vi "Test DAQmx Digitizer.vi"() -> ()   [LabVIEW 2015]
uses:
  Instruments/Pulse Driver/Pusle Driver Configuration.ctl
  DAQmx Digitizer.lvclass
  Instruments/Pulse Driver/Pulse Driver.lvclass/Pulse Driver.ctl
  Instruments/Pulse Driver/Write tdms file.vi
  Instruments/Pulse Driver/Write User Configuration.vi
panel:
  in  "User Configuration":T1={"Pre-trigger duration"=0.01, "Post-trigger duration"=0.1, "Rate"=1000000.0, "Ranges"=[10.0], "Re-name channels"=[], "Active channels"="0:1", "External clock"=FALSE} {"Rate" format="%#_6pHz"; "Post-trigger duration" format="%#_6ps"; "Pre-trigger duration" format="%#_6ps"; "Ranges" format="%#_6pV"}
  in  "File Path Control":path=path "D:/Data/test_daqmx.tdms"
  in  "Stop Button":bool
  out "Availiable Samples":u32=110000
  out "Finished":bool=TRUE
  out "Armed":bool
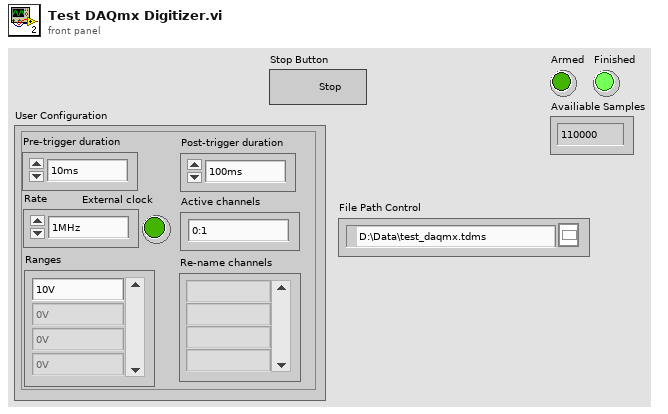
[diagram p1: front panel]
types:
  T1 = typedef "Pusle Driver Configuration.ctl" = cluster{"Pre-trigger duration":dbl, "Post-trigger duration":dbl, "Rate":dbl, "Ranges":dbl[], "Re-name channels":string[], "Active channels":string, "External clock":bool}
  T2 = enum16{"open", "open or create", "create or replace", "create", "open (read-only)"}
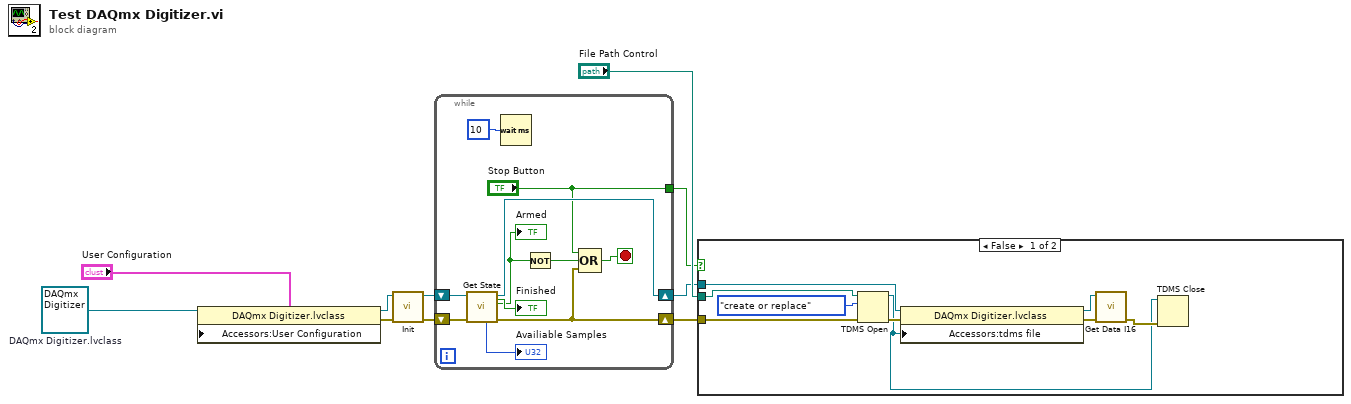
[diagram p0: block diagram]
diagram:
  w10 = refnum<class "DAQmx Digitizer.lvclass"> refnum  # DAQmx Digitizer.lvclass
  n1 = property class="DAQmx Digitizer.lvclass"(reference=w10, "Accessors:User Configuration"="User Configuration") -> (reference out=w9:refnum<class "DAQmx Digitizer.lvclass">, error out=w8:errorcluster)  [unwired: 1 in]
  n2 = call-dynamic "Init.vi"("error in (no error)"=w8, "Pulse Driver in"=w9) -> ("error out"=w6:errorcluster, "Pulse Driver out"=w7:refnum<class "DAQmx Digitizer.lvclass">)  [unwired: 8 in]
  n3 = while {
    shift-right: [w11] -> w5
    shift-left: w6 -> [w20]
    shift-right: [w13] -> w3
    shift-left: w7 -> [w21]
    tunnel: ["Stop Button"] -> w2
    stop <- w16 stop-if-true
    n4 = call-dynamic "Get State.vi"("error in (no error)"=w20, "DAQmx Digitizer in"=w21) -> ("error out"=w11:errorcluster, "Armed"=w15:bool, "DAQmx Digitizer out"=w13:refnum<class "DAQmx Digitizer.lvclass">, "Availiable Samples"=→"Availiable Samples":u32, "Finished"=→"Finished":bool)  [unwired: 4 in, 1 out]
    "Armed" <- w15
    n5 = Wait (ms)(milliseconds to wait=u32 10) -> ()  [unwired: 1 out]
    n6 = Not(x=w15) -> (.not. x?=w14:bool)
    n7 = Compound Arithmetic op=OR("Stop Button", w14, w11) -> (w16:bool)
  }
  n8 = case shown="False" w2 {
    tunnel: w5 -> [w30 _]
    tunnel: "File Path Control" -> [w29 _]
    tunnel: w3 -> [w27 _]
    frame False {
      n9 = TDMS Open(8:w30, 10:T2."create or replace" ("operation (0:open)"), 11:w29) -> (0:w25:errorcluster, 3:w22:refnum<k34>)  [unwired: 4 in]
      n10 = property class="DAQmx Digitizer.lvclass"(reference=w27, error in=w25, "Accessors:tdms file"=w22) -> (reference out=w26:refnum<class "DAQmx Digitizer.lvclass">, error out=w24:errorcluster)
      n11 = call-dynamic "Get Data I16.vi"("error in (no error)"=w24, "DAQmx Digitizer in"=w26) -> ("error out"=w23:errorcluster)  [unwired: 5 in, 4 out]
      n12 = TDMS Close(8:w23, 11:w22) -> ()  [unwired: 2 out]
    }
    frame True {
    }
  }
